vi "Draw Rectangle Helper.vi"(4 "Vision Instrumentation":T3={"Draw Boxes"=TRUE, "Draw Scores"=FALSE, "Draw Lines"=TRUE, "Draw Line Angles"=FALSE, "Draw Targets"=TRUE, "Draw Compound Crosshair"=TRUE, "Draw Center Line"=TRUE}, 5 "Diamond Targets":T6[](array[typedef]), 6 "Image Size":cluster{i32, i32}, 7 "Lines":T8[][](array[typedef]), 8 "Targetting Output":T2, 9 "Targets":T10[](array[typedef]), 10 "Score Limits":dbl[](array[numeric]), 11 "Refnum in":T11) -> (3 "Refnum out":T11)   [LabVIEW 2011]
uses:
  <vilib>/vision/Image Controls.llb/IMAQ Image.ctl
  Target Data.ctl
  Line.ctl
  Direction.ctl
  Line Confidence.ctl
  Diamond Target Output.ctl
  Rectangle Position.ctl
  Target Confidence.ctl
  Vision Instrumentation Control.ctl
  Camera State.ctl
panel:
  in  "Camera State Colors":u32[](array[colorbox])=[16711680, 16759314, 16722675, 6618880, 16860]
  in  "Camera State":T1
  in  "Est. Position":T4
  in  "Direction Bias":cluster{"X":dbl, "Y":dbl}[](array[cluster])=[{"X"=0.0, "Y"=8.0}, {"X"=8.0, "Y"=8.0}, {"X"=8.0, "Y"=0.0}, {"X"=8.0, "Y"=-8.0}, {"X"=0.0, "Y"=-8.0}, {"X"=-8.0, "Y"=-8.0}, {"X"=-8.0, "Y"=0.0}, {"X"=-8.0, "Y"=8.0}, {"X"=0.0, "Y"=0.0}]
  in  "Direction":T5
  in  "Line Colors":u32[](array[colorbox])=[16711680, 16756778, 7274329, 5898223, 4349695, 11539199, 16728807, 16774745]
  in  "Crosshair Size":dbl=8.0
  in  "Crosshair Colors":u32[](array[colorbox])=[16711680, 6618880, 16860, 1245142, 16711930]
  # "Note: I use this VI to customize the interface of the existing Draw Rect VI"
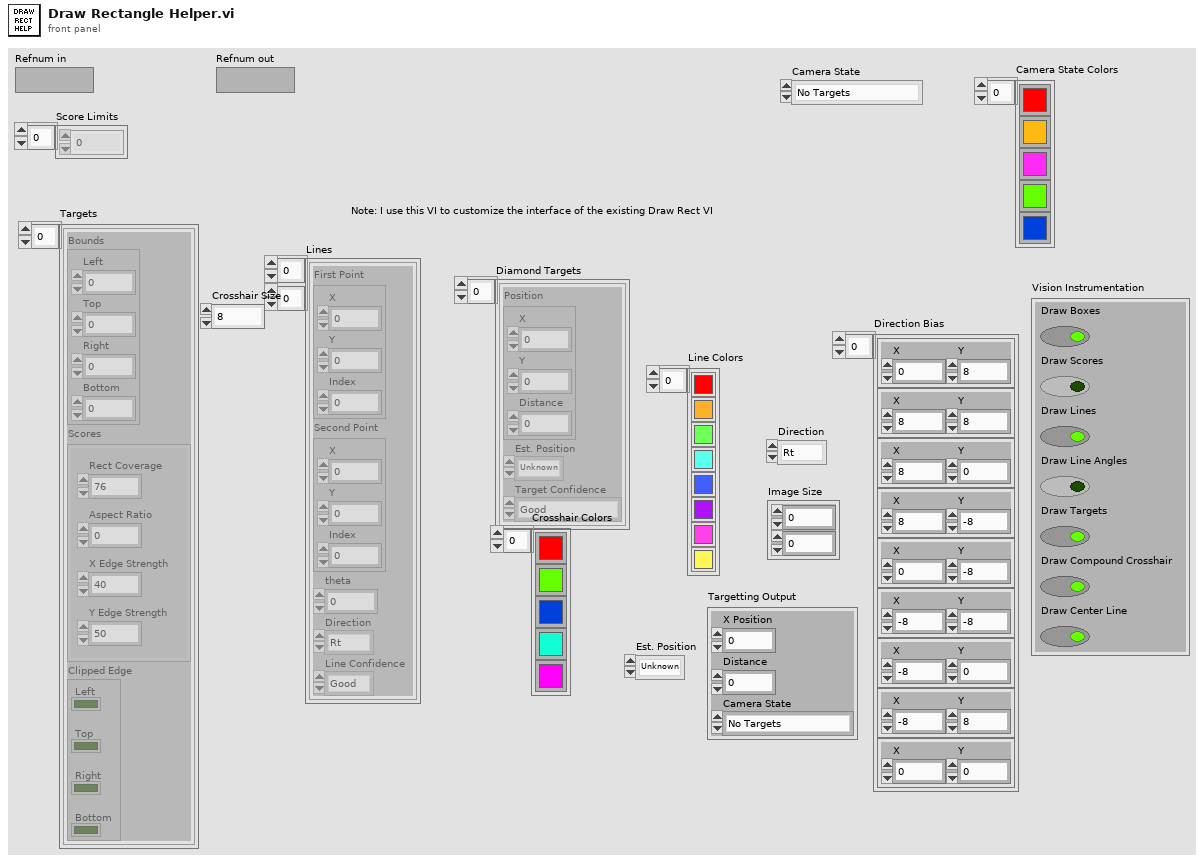
[diagram p1: front panel]
types:
  T1 = typedef "Camera State.ctl" = enum16{"No Targets", "Low Confidence", "Medium Confidence", "High Confidence", "Camera Error"}
  T2 = cluster{"X Position":dbl, "Distance":dbl, "Camera State":T1}
  T3 = typedef "Vision Instrumentation Control.ctl" = cluster{"Draw Boxes":bool, "Draw Scores":bool, "Draw Lines":bool, "Draw Line Angles":bool, "Draw Targets":bool, "Draw Compound Crosshair":bool, "Draw Center Line":bool}
  T4 = typedef "Rectangle Position.ctl" = enum16{"Unknown", "Top", "Right", "Left", "Bottom"}
  T5 = typedef "Direction.ctl" = enum16{"Rt", "Rt-Up", "Up", "Lt-Up", "Lt", "Lt-Dn", "Dn", "Rt-Dn", "Unknown"}
  T6 = typedef "Diamond Target Output.ctl" = cluster{"Position":cluster{"X":dbl, "Y":dbl, "Distance":dbl}, "Est. Position":T4, "Target Confidence":T7}
  T7 = typedef "Target Confidence.ctl" = enum16{"Good", "Good-Clipped Y", "Marginal-Clipped X"}
  T8 = typedef "Line.ctl" = cluster{"First Point":cluster{"X":dbl, "Y":dbl, "Index":dbl}, "Second Point":cluster{"X":dbl, "Y":dbl, "Index":dbl}, "theta":dbl, "Direction":T5, "Line Confidence":T9}
  T9 = typedef "Line Confidence.ctl" = enum16{"Good", "Bad"}
  T10 = typedef "Target Data.ctl" = cluster{"Bounds":cluster{"Left":dbl, "Top":dbl, "Right":dbl, "Bottom":dbl}, "Scores":cluster{"Rect Coverage":dbl, "Aspect Ratio":dbl, "X Edge Strength":dbl, "Y Edge Strength":dbl}, "Clipped Edge":cluster{"Left":bool, "Top":bool, "Right":bool, "Bottom":bool}}
  T11 = typedef "IMAQ Image.ctl" = refnum<image>
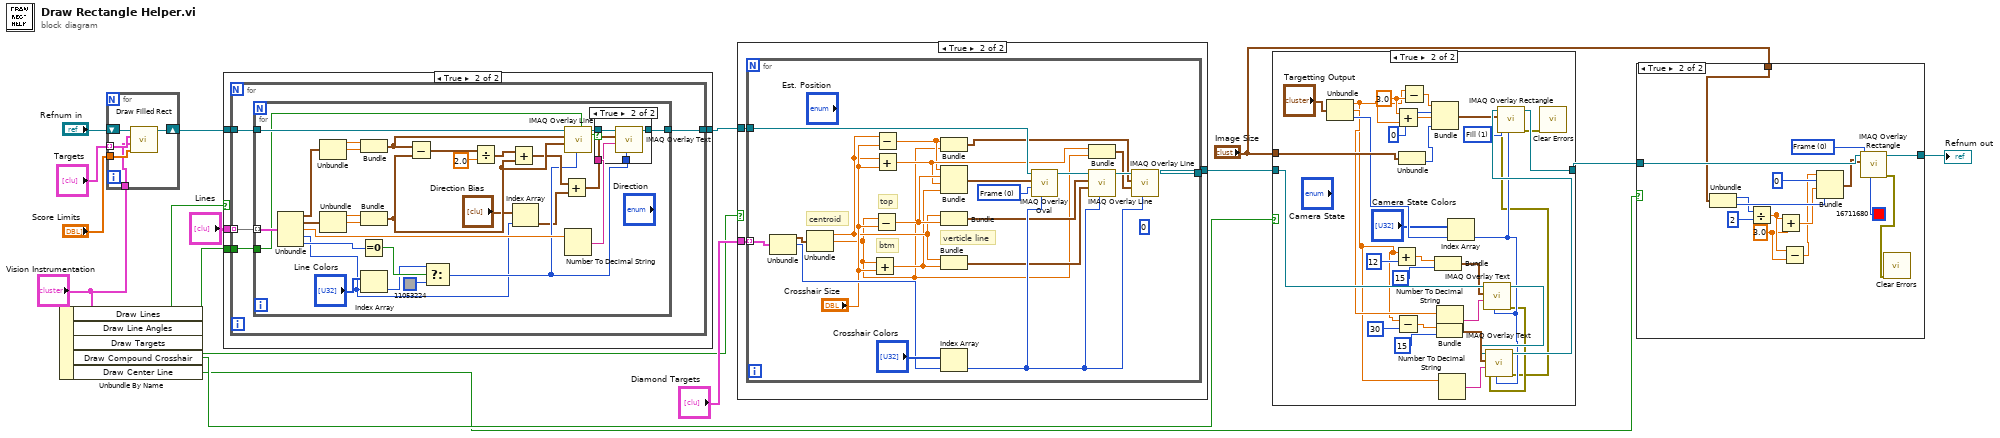
[diagram p0: block diagram]
diagram:
  n1 = Unbundle By Name("Vision Instrumentation") -> ("Draw Lines"=w9:bool, "Draw Line Angles"=w8:bool, "Draw Targets"=w7:bool, "Draw Compound Crosshair"=w5:bool, "Draw Center Line"=w1:bool)
  n2 = for {
    shift-right: [w21] -> w14
    shift-left: "Refnum in" -> [w22]
    tunnel: "Targets" -> [w19] mode=indexing
    tunnel: "Score Limits" -> [w20]
    tunnel: "Vision Instrumentation" -> [w18]
    n3 = call "Draw Filled Rect.vi"("Limits"=w20, "Vision Instrumentation"=w18, "Target Data"=w19, "image in"=w22) -> ("image out"=w21:T11)  [unwired: 7 in]
  }
  n4 = case shown="True" w9 {
    tunnel: w14 -> [w23 w27]
    tunnel: "Lines" -> [_ w26]
    tunnel: [w23 w25] -> w12
    tunnel: w8 -> [_ w24]
    frame False {
    }
    frame True {
      n5 = for {
        tunnel: w27 -> [w31]
        tunnel: w26 -> [w30] mode=indexing
        tunnel: [w29] -> w25
        tunnel: w24 -> [w28]
        n6 = for {
          tunnel: w31 -> [w60]
          tunnel: w30 -> [w59] mode=indexing
          tunnel: [w41] -> w29
          tunnel: w28 -> [w32]
          n7 = Unbundle(w59) -> ("First Point"=w58:cluster{"X":dbl, "Y":dbl, "Index":dbl}, "Second Point"=w55:cluster{"X":dbl, "Y":dbl, "Index":dbl}, "theta"=w38:dbl, "Direction"=w34:T5, "Line Confidence"=w52:T9)
          n8 = Unbundle(w58) -> ("X"=w57:dbl, "Y"=w56:dbl)  [unwired: 1 out]
          n9 = Unbundle(w55) -> ("X"=w54:dbl, "Y"=w53:dbl)  [unwired: 1 out]
          n10 = Equal To 0?(x=w52) -> (x = 0?=w51:bool)
          n11 = Bundle("X"=w57, "Y"=w56) -> (w47:cluster{"X":dbl, "Y":dbl})  [unwired: 1 in]
          n12 = Bundle("X"=w54, "Y"=w53) -> (w43:cluster{"X":dbl, "Y":dbl})  [unwired: 1 in]
          n13 = Index Array(array="Line Colors", index=w34) -> (element=w48:u32)
          n14 = Subtract(x=w47, y=w43) -> (x-y=w46:cluster{"X":dbl, "Y":dbl})
          n15 = Select(t=w48, s=w51, f=u32 11053224 ("Color")) -> (s? t:f=w36:u32)
          n16 = Divide(x=w46, y=2.0) -> (x/y=w44:cluster{"X":dbl, "Y":dbl})
          n17 = Add(x=w44, y=w43) -> (x+y=w39:cluster{"X":dbl, "Y":dbl})
          n18 = Index Array(array="Direction Bias", index=w34) -> (element=w33:cluster{"X":dbl, "Y":dbl})
          n19 = Add(x=w39, y=w33) -> (x+y=w40:cluster{"X":dbl, "Y":dbl})
          n20 = call "IMAQ Overlay Line"("Color"=w36, "End Point"=w43, "Start Point"=w47, "Image"=w60) -> ("Image Out"=w42:T11)  [unwired: 6 in, 1 out]
          n21 = Number To Decimal String(number=w38) -> (decimal integer string=w37:string)  [unwired: 1 in]
          n22 = case shown="True" w32 {
            tunnel: w42 -> [w61 w66]
            tunnel: [w61 w65] -> w41
            tunnel: w40 -> [_ w64]
            tunnel: w37 -> [_ w63]
            tunnel: w36 -> [_ w62]
            frame False {
            }
            frame True {
              n23 = call "IMAQ Overlay Text"("Text Color (black)"=w62, "String"=w63, "Origin"=w64, "Image"=w66) -> ("Image Out"=w65:T11)  [unwired: 6 in, 1 out]
            }
          }
        }
      }
    }
  }
  n24 = case shown="True" w7 {
    tunnel: w12 -> [w67 w70]
    tunnel: "Diamond Targets" -> [_ w69]
    tunnel: [w67 w68] -> w6
    frame False {
    }
    frame True {
      n25 = for {
        tunnel: w70 -> [w89]
        tunnel: w69 -> [w92] mode=indexing
        tunnel: [w88] -> w68
        (unwired) 0 ("index")
        w83 = u32 0 items=["Frame", "Fill"] ("Drawing Mode (Frame)")
        # "verticle line"
        # "btm"
        # "top"
        # "centroid"
        n26 = Unbundle(w92) -> ("Position"=w84:cluster{"X":dbl, "Y":dbl, "Distance":dbl}, "Est. Position"=w86:T4)  [unwired: 1 out]
        n27 = Unbundle(w84) -> ("X"=w78:dbl, "Y"=w71:dbl)  [unwired: 1 out]
        n28 = Add(x=w71, y="Crosshair Size") -> (x+y=w77:dbl)
        n29 = Subtract(x=w71, y="Crosshair Size") -> (x-y=w79:dbl)
        n30 = Subtract(x=w78, y="Crosshair Size") -> (x-y=w72:dbl)
        n31 = Add(x=w78, y="Crosshair Size") -> (x+y=w73:dbl)
        n32 = Bundle(w72, "Y"=w71) -> (w75:cluster{dbl, "Y":dbl})  [unwired: 1 in]
        n33 = Bundle(w72, w79, w73, w77) -> (w85:cluster{dbl, dbl, dbl, dbl})  [unwired: 1 in]
        n34 = Bundle("X"=w78, w79) -> (w80:cluster{"X":dbl, dbl})  [unwired: 1 in]
        n35 = Bundle("X"=w78, w77) -> (w76:cluster{"X":dbl, dbl})  [unwired: 1 in]
        n36 = Index Array(array="Crosshair Colors", index=w86) -> (element=w82:u32)
        n37 = call "IMAQ Overlay Oval"("Color"=w82, "Drawing Mode (Frame)"=w83, "Bounding Rectangle"=w85, "Image"=w89) -> ("Image Out"=w90:T11)  [unwired: 6 in, 1 out]
        n38 = Bundle(w73, "Y"=w71) -> (w74:cluster{dbl, "Y":dbl})  [unwired: 1 in]
        n39 = call "IMAQ Overlay Line"("Color"=w82, "End Point"=w76, "Start Point"=w80, "Image"=w90) -> ("Image Out"=w91:T11)  [unwired: 6 in, 1 out]
        n40 = call "IMAQ Overlay Line"("Color"=w82, "End Point"=w74, "Start Point"=w75, "Image"=w91) -> ("Image Out"=w88:T11)  [unwired: 6 in, 1 out]
      }
    }
  }
  n41 = case shown="True" w5 {
    tunnel: [w93 w106] -> w4
    tunnel: w6 -> [w93 w120]
    tunnel: "Image Size" -> [_ w124]
    frame False {
    }
    frame True {
      w97 = u32 1 items=["Frame", "Fill", "Highlight"] ("Drawing Mode (Frame)")
      w100 = 3.0 ("y")
      n42 = Unbundle("Targetting Output") -> ("X Position"=w99:dbl, "Distance"=w115:dbl, "Camera State"=w122:T1)
      n43 = Add(x=w99, y=12) -> (x+y=w117:dbl)
      n44 = Add(x=w100, y=w99) -> (x+y=w101:dbl)
      n45 = Subtract(x=w99, y=30) -> (x-y=w111:dbl)
      n46 = Unbundle(w124) -> (w104:i32)  [unwired: 1 out]
      n47 = Subtract(x=w99, y=w100) -> (x-y=w102:dbl)
      n48 = Bundle(w102, 0, w101, w104) -> (w98:cluster{dbl, i32, dbl, i32})  [unwired: 1 in]
      n49 = Bundle(w117, 15) -> (w119:cluster{dbl, i32})  [unwired: 1 in]
      n50 = Bundle(w111, 15) -> (w113:cluster{dbl, i32})  [unwired: 1 in]
      n51 = Number To Decimal String(number=w115) -> (decimal integer string=w114:string)  [unwired: 1 in]
      n52 = Number To Decimal String(number=w99) -> (decimal integer string=w109:string)  [unwired: 1 in]
      n53 = Index Array(array="Camera State Colors", index=w122) -> (element=w105:u32)
      n54 = call "IMAQ Overlay Text"("Text Color (black)"=w105, "String"=w114, "Origin"=w119, "Image"=w120) -> ("error out"=w96:errorcluster, "Image Out"=w108:T11)  [unwired: 6 in]
      n55 = call "IMAQ Overlay Text"("Text Color (black)"=w105, "error in (no error)"=w96, "String"=w109, "Origin"=w113, "Image"=w108) -> ("error out"=w95:errorcluster, "Image Out"=w107:T11)  [unwired: 5 in]
      n56 = call "IMAQ Overlay Rectangle"("Color"=w105, "error in (no error)"=w95, "Drawing Mode (Frame)"=w97, "Rectangle"=w98, "Image"=w107) -> ("error out"=w94:errorcluster, "Image Out"=w106:T11)  [unwired: 5 in]
      n57 = call <vilib>:"Clear Errors.vi"("error in (no error)"=w94) -> ()  [unwired: 6 in, 1 out]
    }
  }
  n58 = case shown="True" w1 {
    tunnel: w4 -> [w125 w140]
    tunnel: [w125 w139] -> w3
    tunnel: "Image Size" -> [_ w135]
    frame False {
    }
    frame True {
      w127 = u32 0 items=["Frame", "Fill", "Highlight"] ("Drawing Mode (Frame)")
      w129 = 3.0 ("y")
      n59 = Unbundle(w135) -> (w133:i32, w134:i32)
      n60 = Divide(x=w133, y=2) -> (x/y=w130:dbl)
      n61 = Add(x=w130, y=w129) -> (x+y=w131:dbl)
      n62 = Subtract(x=w130, y=w129) -> (x-y=w128:dbl)
      n63 = Bundle(w128, 0, w131, w134) -> (w138:cluster{dbl, i32, dbl, i32})  [unwired: 1 in]
      n64 = call "IMAQ Overlay Rectangle"("Color"=u32 16711680, "Drawing Mode (Frame)"=w127, "Rectangle"=w138, "Image"=w140) -> ("error out"=w126:errorcluster, "Image Out"=w139:T11)  [unwired: 6 in]
      n65 = call <vilib>:"Clear Errors.vi"("error in (no error)"=w126) -> ()  [unwired: 6 in, 1 out]
    }
  }
  "Refnum out" <- w3
